vi "validate line configuration.vi"(7 "Profibus Module configuration":refnum<class "Profibus Module configuration.lvclass">, 11 "line in":T1) -> (1 "valid?":bool, 3 "line out":T1)   [LabVIEW 2013, in "Profibus Module editor node.lvclass"]
uses:
  Profibus Module editor node.lvclass
  table line.ctl
  channel/Profibus channel.lvclass
  configuration/Profibus Module configuration.lvclass
  <vilib>/NI/Tag Bus Module Framework/channel/channel classification.ctl
  <vilib>/NI/Tag Bus/tag/tag descriptor.lvclass/tag descriptor.ctl
  channel/Profibus channel.lvclass/Profibus channel.ctl
  <vilib>/NI/Tag Bus Module Framework/channel/TBM channel.lvclass/TBM channel.ctl
  <vilib>/NI/Tag Bus/tag/read tag name.vi
  <vilib>/NI/Tag Bus/tag/read data type.vi
  channel/Read bit.vi
  <vilib>/NI/Tag Bus Module Framework/channel/Read channel classification.vi
  <vilib>/NI/Tag Bus Module Framework/channel/TBM channel.lvclass
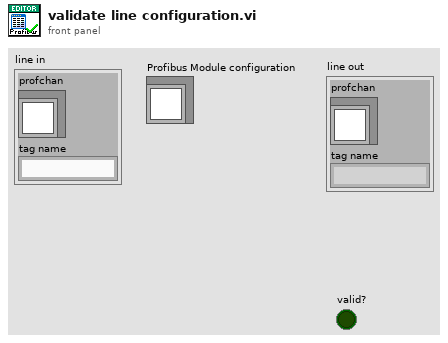
[diagram p1: front panel]
types:
  T1 = typedef "Profibus Module editor node.lvclass/table line.ctl" = cluster{"profchan":refnum<class "Profibus channel.lvclass">, "tag name":string}
  T2 = typedef "TBM channel.lvclass/channel classification.ctl" = enum16{"input data", "output data", "processing parameter", "processing result"}
  T3 = typedef "tag bus.lvlib/tag descriptor.lvclass/Data Type.ctl" = enum16{"Double", "Single", "I64", "I32", "I16", "I8", "U64", "U32", "U16", "U8", "Boolean", "String", "Array of Double", "Array of Single", "Array of I64", "Array of I32", "Array of I16", "Array of I8", "Array of U64", "Array of U32", "Array of U16", "Array of U8", "Array of Boolean", "Array of String"}
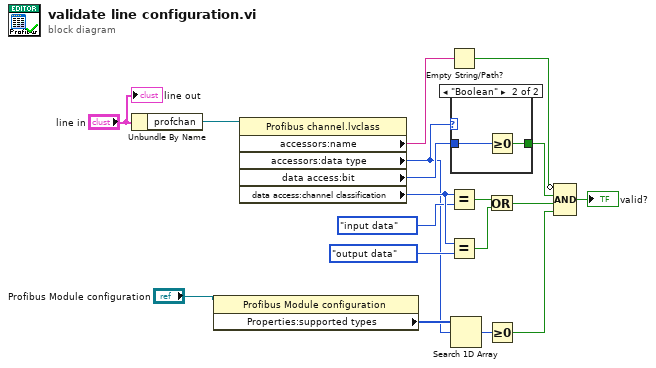
[diagram p0: block diagram]
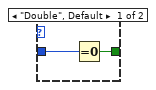
[diagram p2: hidden frame]
diagram:
  n1 = Unbundle By Name("line in") -> ("profchan"=w17:refnum<class "Profibus channel.lvclass">)
  n2 = property class="Profibus Module configuration"(reference="Profibus Module configuration") -> ("Properties:supported types"=w4:T3[])  [unwired: 1 in, 2 out]
  n3 = property class="Profibus channel.lvclass"(reference=w17) -> ("accessors:name"=w16:string, "accessors:data type"=w1:T3, "data access:bit"=w15:i32, "data access:channel classification"=w11:T2)  [unwired: 1 in, 2 out]
  n4 = Empty String/Path?(string/path=w16) -> (empty?=w14:bool)
  n5 = Equal?(x=w11, y=channel_classification."input data") -> (x = y?=w7:bool)
  n6 = Equal?(x=w11, y=channel_classification."output data") -> (x = y?=w8:bool)
  n7 = case shown="\"Boolean\"" w1 {
    tunnel: w15 -> [w20 w22]
    tunnel: [w19 w21] -> w12
    frame "Double", Default {
      n8 = Equal To 0?(x=w20) -> (x = 0?=w19:bool)
    }
    frame "Boolean" {
      n9 = Greater Or Equal To 0?(x=w22) -> (x >= 0?=w21:bool)
    }
  }
  n10 = Search 1D Array(1D array=w4, element=w1) -> (index of element=w3:i32)  [unwired: 1 in]
  n11 = Or(x=w7, y=w8) -> (x .or. y?=w6:bool)
  n12 = Greater Or Equal To 0?(x=w3) -> (x >= 0?=w2:bool)
  n13 = Compound Arithmetic op=AND(invert w14, w12, w6, w2) -> (→"valid?":bool)
  "line out" <- "line in"
